vi "test.vi"() -> ()   [LabVIEW 2016]
uses:
  Source/JSON Variant Support/JSON Variant Support.lvclass
panel:
  out "error out":errorcluster
  out "data":cluster{"String":string}
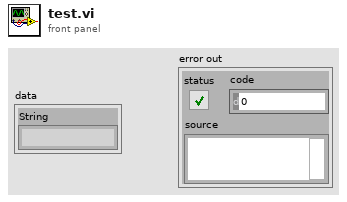
[diagram p1: front panel]
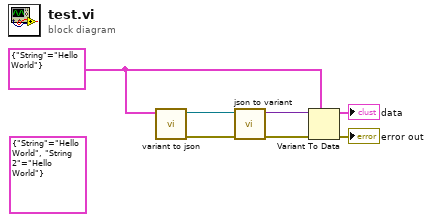
[diagram p0: block diagram]
diagram:
  (unwired) cluster{"String":string, "String 2":string} {"String"="Hello World", "String 2"="Hello World"}
  w5 = cluster{"String":string} {"String"="Hello World"}
  n1 = call "variant to json.vi"("Variant"=w5) -> ("error out"=w3:errorcluster, "JSON Value"=w7:refnum<class "JSON Value.lvclass">)  [unwired: 9 in]
  n2 = call "json to variant.vi"("error in (no error)"=w3, "JSON Value"=w7) -> ("error out"=w2:errorcluster, "Variant"=w4:variant)  [unwired: 8 in]
  n3 = Variant To Data(error in=w2, type=w5, Variant=w4) -> (data=→"data":cluster{"String":string}, error out=→"error out":errorcluster)
